vi "Draw Circle.vi"(1 "radius":dbl, 2 "Pos XY":dbl[](array[numeric])) -> (0 "Bound out":T1)   [LabVIEW 2016]
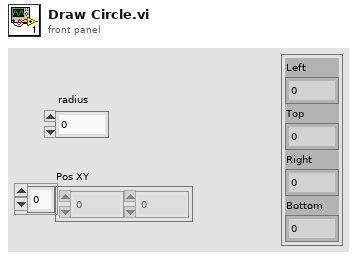
[diagram p1: front panel]
types:
  T1 = cluster{"Left":i32, "Top":i32, "Right":i32, "Bottom":i32}
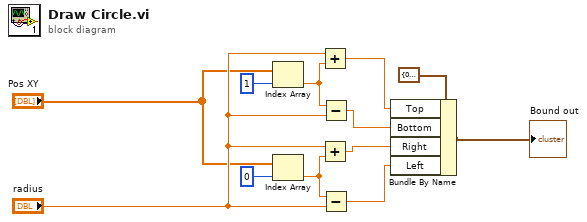
[diagram p0: block diagram]
diagram:
  n1 = Index Array(array="Pos XY", index=1 ("索引")) -> (element=w9:dbl)
  n2 = Index Array(array="Pos XY", index=0 ("索引")) -> (element=w8:dbl)
  n3 = Add(x="radius", y=w9) -> (x+y=w5:dbl)
  n4 = Add(x="radius", y=w8) -> (x+y=w3:dbl)
  n5 = Subtract(x=w9, y="radius") -> (x-y=w4:dbl)
  n6 = Subtract(x=w8, y="radius") -> (x-y=w2:dbl)
  n7 = Bundle By Name(cluster=T1 {"Left"=0, "Top"=0, "Right"=0, "Bottom"=0} ("Bounding Rectangle"), "Top"=w5, "Bottom"=w4, "Right"=w3, "Left"=w2) -> (→"Bound out":T1)
